vi "CreateLogger.vi"(7 "Level":T1, 8 "error in (no error)":errorcluster, 9 "log-file name (without suffix)":string="LogFile", 10 "path of log file\n(default: folder of this vi)":path, 11 "Handler Name":string="example logger handler") -> (0 "error out":errorcluster, 3 "log-file path":path)   [LabVIEW 2023]
uses:
  <vilib>/Hampel Software Engineering/HSE Logger/LogLevel.ctl
  <vilib>/Hampel Software Engineering/HSE Logger/Handler/FileHandler/FileHandler.lvclass
  C:/Program Files (x86)/National Instruments/LabVIEW 2023/vi.lib/Hampel Software Engineering/HSE Logger/Handler/Handler.lvclass
  <vilib>/Hampel Software Engineering/HSE Logger/hse-logger.lvlib
  <vilib>/Hampel Software Engineering/HSE Logger/Formatter/Formatter.lvclass
panel:
  # "Connector Pane"
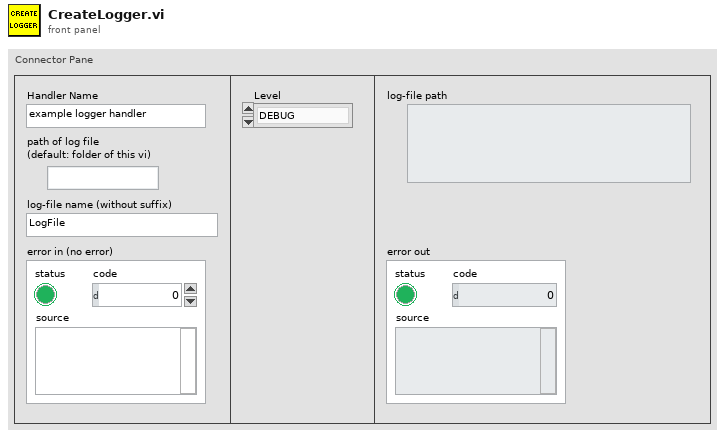
[diagram p1: front panel]
types:
  T1 = typedef "hse-logger.lvlib/LogLevel.ctl" = enum16{"DEBUG", "INFO", "WARNING", "ERROR", "CRITICAL"}
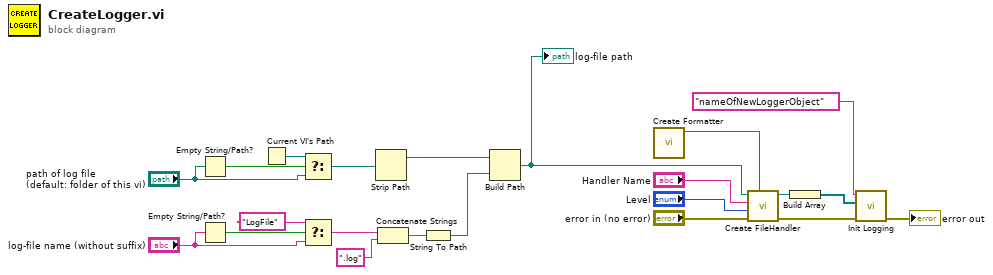
[diagram p0: block diagram]
diagram:
  n1 = Empty String/Path?(string/path="path of log file\n(default: folder of this vi)") -> (empty?=w17:bool)
  n2 = Empty String/Path?(string/path="log-file name (without suffix)") -> (empty?=w13:bool)
  n3 = Current VI's Path() -> (path=w16:path)
  n4 = Select(t=w16, s=w17, f="path of log file\n(default: folder of this vi)") -> (s? t:f=w14:path)
  n5 = Select(t="LogFile", s=w13, f="log-file name (without suffix)") -> (s? t:f=w10:string)
  n6 = Strip Path(path=w14) -> (stripped path=w21:path)  [unwired: 1 out]
  n7 = Concatenate Strings(w10, ".log") -> (w19:string)
  n8 = String To Path(string=w19) -> (path=w18:path)
  n9 = Build Path(base path=w21, name or relative path=w18) -> (appended path=w22:path)
  "log-file path" <- w22
  n10 = call <vilib>:"Create Formatter.vi"() -> ("Formatter out"=w1:refnum<class "Formatter.lvclass">)  [unwired: 10 in, 1 out]
  n11 = call <vilib>:"Create FileHandler.vi"("Formatter.lvclass"=w1, "error in"="error in (no error)", "Level"="Level", "Name"="Handler Name", "Filepath"=w22) -> ("error out"=w2:errorcluster, "FileHandler out"=w5:refnum<class "FileHandler.lvclass">)  [unwired: 5 in]
  n12 = Build Array(w5) -> (w6:refnum<class "FileHandler.lvclass">[])
  n13 = call <vilib>:"Init Logging.vi"("error in"=w2, "Handlers"=w6, "Name"="nameOfNewLoggerObject") -> ("error out"=→"error out":errorcluster)  [unwired: 8 in]
